vi "_Random Change Flag.vi"() -> (1 "Random Change Flag":u64)   [LabVIEW 2017, in "INI-Static-Variable-Support.lvlib"]
uses:
  INI-Static-Variable-Support.lvlib
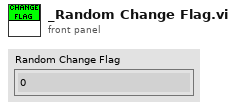
[diagram p1: front panel]
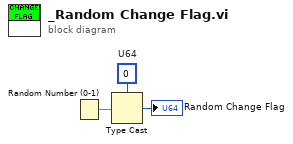
[diagram p0: block diagram]
diagram:
  w2 = u64 0  # U64
  n1 = Random Number (0-1)() -> (number: 0 to 1=w3:dbl)
  n2 = Type Cast(type=w2, x=w3) -> (*(type *) &x=→"Random Change Flag":u64)
